vi "c2fnew(SubVI).vi"(1 "Boolean":bool, 2 "Degrees C":dbl) -> (0 "Numeric":dbl)   [LabVIEW 2015]
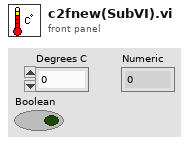
[diagram p1: front panel]
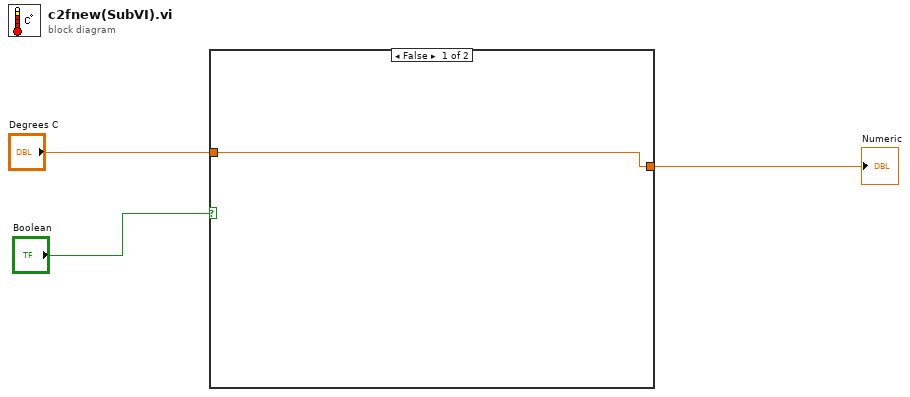
[diagram p0: block diagram]
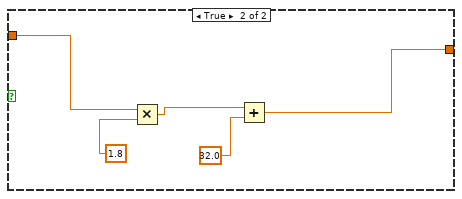
[diagram p2: hidden frame]
diagram:
  n1 = case shown="False" "Boolean" {
    tunnel: [w4 w9] -> w3
    tunnel: "Degrees C" -> [w4 w5]
    frame False {
    }
    frame True {
      n2 = Multiply(x=w5, y=1.8) -> (x*y=w7:dbl)
      n3 = Add(x=w7, y=32.0) -> (x+y=w9:dbl)
    }
  }
  "Numeric" <- w3
